vi "Host Main.vi"() -> ()   [LabVIEW 2021]
doc: "This application launches and executes the Tag Bus Data framework configuration for the specified target alias. This is a simple example of the framework API functions, but may also be a suitable starting point for a Host UI or Thick Client that is running a local version of the framework."
uses:
  <vilib>/NI/Module Execution Interface/Engine Runtime/Execution States.ctl
  <vilib>/NI/Module Execution Interface/Engine Runtime/Fault.ctl
  <vilib>/NI/Tag Bus Module Framework/runtime/error classification.ctl
  <vilib>/userdefined/High Color/nirio_resource_hc.ctl
  <vilib>/NI/Module Execution Interface/Engine Runtime/Engine Runtime Interface.lvclass
  <vilib>/NI/DCAF/Tag Editor Core/Framework Configuration Classes/target runtime/PL_Target Runtime.lvclass
  <vilib>/NI/Tag Bus Module Framework/FPGA manager/FPGA manager.lvlib
  <vilib>/rvi/interface/nirviOpenFPGA/nirviOpenFPGA.xnode
  <vilib>/NI/Tag Bus Module Framework/FPGA manager/methods.ctl
  <vilib>/NI/Tag Bus Module Framework/runtime/TBM module execution interface.lvclass
panel:
  in  "configuration file path":path=path "C:/Documentation/Trunk/Getting Started Material/Hands On/Hands-On_3/Excercises/Multiplexer/Multiplexer.pcfg"
  in  "target alias":string="PC"
  out "engine status":T4(array[cluster])
  in  "stop":bool
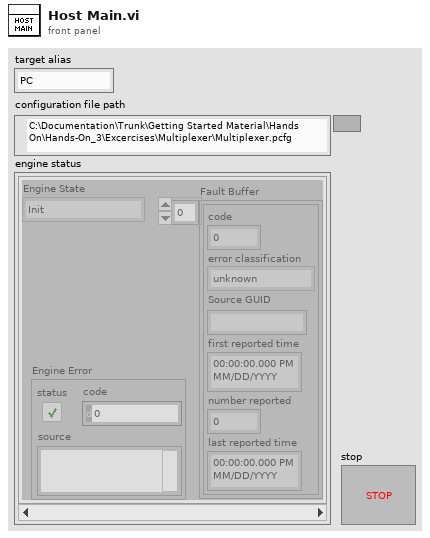
[diagram p1: front panel]
types:
  T1 = typedef "Engine Runtime Interface.lvclass/Execution States.ctl" = enum16{"Init", "Pre-Operational", "Safe-Operational", "Operational", "Stopped"}
  T2 = typedef "Engine Runtime Interface.lvclass/Fault.ctl" = cluster{"code":i32, "error classification":T3, "Source GUID":string, "first reported time":timestamp, "number reported":u32, "last reported time":timestamp}
  T3 = typedef "TBM module execution interface.lvclass/error classification.ctl" = enum16{"unknown", "none", "trivial", "recoverable", "critical"}
  T4 = cluster{"Engine State":T1, "Fault Buffer":T2[], "Engine Error":errorcluster}[]
  T5 = typedef "FPGA manager.lvlib/methods.ctl" = enum16{"initialize bitfile", "cache bitfile", "locate bitfile", "close bitfile", "clear manager"}
  T6 = typedef "nirio_resource_hc.ctl" = tag
  T7 = cluster{"Engine State":T1, "Fault Buffer":T2[], "Engine Error":errorcluster}
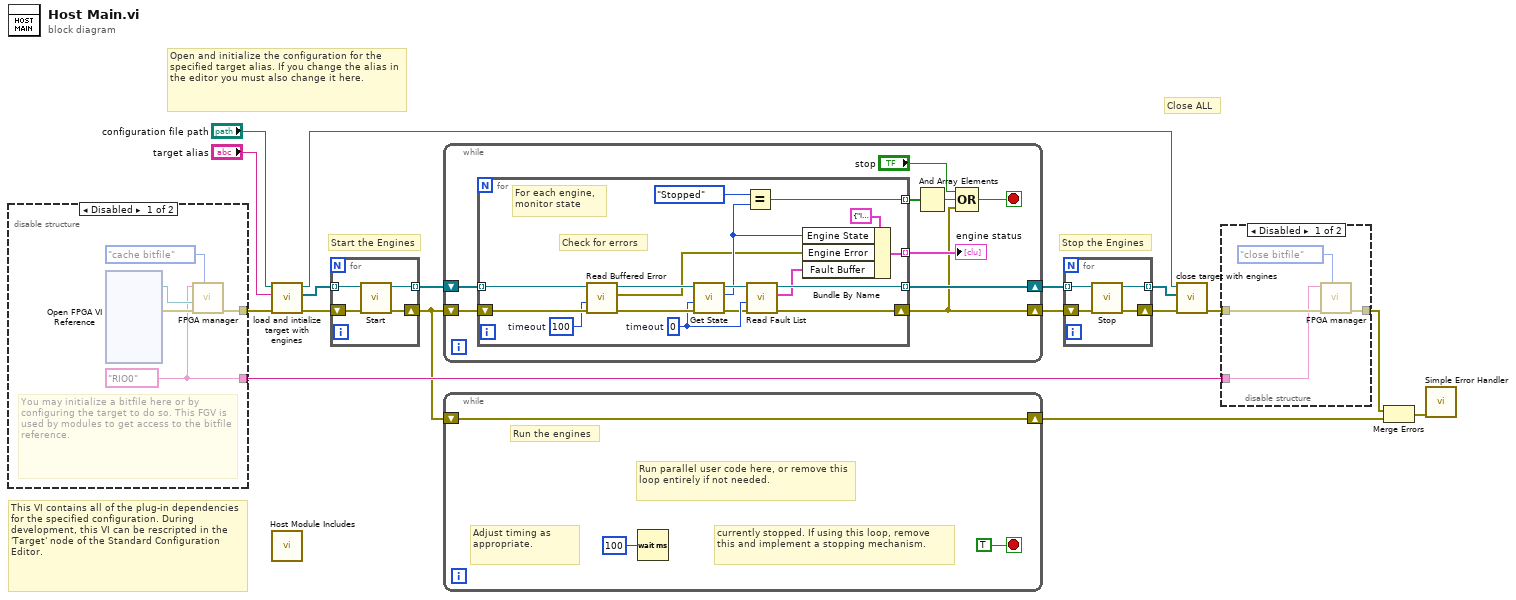
[diagram p0: block diagram]
diagram:
  # "Start the Engines"
  # "Open and initialize the configuration for the specified target alias. If you change the alias in the editor you must also change it here."
  # "Close ALL"
  # "Stop the Engines"
  # "This VI contains all of the plug-in dependencies for the specified configuration. During development, this VI can be rescripted in the 'Target' node of the Standard Configuration Editor."
  # "Run the engines"
  n1 = disable-structure shown="Disabled" {
    disable-tunnel: [w22 _] -> w7
    disable-tunnel: [w18 _] -> w6
    frame Disabled {
      w18 = T6 "RIO0" ("RIO resource")
      # "You may initialize a bitfile here or by configuring the target to do so. This FGV is used by modules to get access to the bitfile reference."
      n2 = xnode "Open FPGA VI Reference"() -> ("FPGA VI Reference Out"=w20:refnum<k20>, "error out"=w21:errorcluster)  [unwired: 2 in]
      n3 = call <vilib>:"FPGA manager.vi"("action"=methods."cache bitfile", "error in"=w21, "bitfile to cache"=w20, "RIO resource"=w18) -> ("error out"=w22:errorcluster)  [unwired: 5 in, 2 out]
    }
    frame Enabled {
    }
  }
  n4 = call <vilib>:"load and intialize target with engines.vi"("error in"=w7, "target alias"="target alias", "file path"="configuration file path") -> ("error out"=w14:errorcluster, "engine runtime interfaces"=w13:refnum<class "Engine Runtime Interface.lvclass">[], "target runtime"=w10:refnum<class "PL_Target Runtime.lvclass">)  [unwired: 6 in]
  n5 = call "Host Module Includes.vi"() -> ()  [unwired: 12 in]
  n6 = for {
    tunnel: [w26] -> w17 mode=indexing
    tunnel: w13 -> [w23] mode=indexing
    shift-right: [w25] -> w5
    shift-left: w14 -> [w24]
    n7 = call-dynamic "Start.vi"("error in"=w24, "Engine Runtime Interface in"=w23) -> ("error out"=w25:errorcluster, "Engine Runtime Interface out"=w26:refnum<class "Engine Runtime Interface.lvclass">)  [unwired: 8 in]
  }
  n8 = while {
    shift-right: [w33] -> w16
    shift-left: w17 -> [w35]
    shift-right: [w27] -> w15
    shift-left: w5 -> [w34]
    stop <- w31 stop-if-true
    n9 = for {
      tunnel: w35 -> [w52] mode=indexing
      tunnel: [w44] -> w33 mode=indexing
      tunnel: [w47] -> w29 mode=indexing
      shift-right: [w43] -> w27
      shift-left: w34 -> [w51]
      tunnel: [w39] -> w30 mode=indexing
      w42 = 0  # timeout
      w46 = 100  # timeout
      # "For each engine, \nmonitor state"
      # "Check for errors"
      n10 = call-dynamic "Read Buffered Error.vi"("error in"=w51, "timeout in ms (0)"=w46, "Engine Runtime Interface in"=w52) -> ("error out"=w49:errorcluster, "Engine Error"=w37:errorcluster, "Engine Runtime Interface out"=w50:refnum<class "Engine Runtime Interface.lvclass">)  [unwired: 6 in]
      n11 = call-dynamic "Get State.vi"("error in"=w49, "timeout (-1)"=w42, "Engine Runtime Interface in"=w50) -> ("error out"=w36:errorcluster, "Engine State"=w41:T1, "Engine Runtime Interface out"=w45:refnum<class "Engine Runtime Interface.lvclass">)  [unwired: 6 in]
      n12 = Equal?(x=Execution_States."Stopped" ("Engine State"), y=w41) -> (x = y?=w47:bool)
      n13 = call-dynamic "Read Fault List.vi"("error in"=w36, "timeout (-1)"=w42, "Engine Runtime Interface in"=w45) -> ("error out"=w43:errorcluster, "faults"=w40:T2[], "Engine Runtime Interface out"=w44:refnum<class "Engine Runtime Interface.lvclass">)  [unwired: 6 in]
      n14 = Bundle By Name(cluster=T7 {"Engine State"=enum."Init", "Fault Buffer"=[], "Engine Error"={"status"=FALSE, "code"=0, "source"=""}}, "Engine State"=w41, "Engine Error"=w37, "Fault Buffer"=w40) -> (w39:T7)
    }
    "engine status" <- w30
    n15 = And Array Elements(Boolean array=w29) -> (logical AND=w28:bool)
    n16 = Compound Arithmetic op=OR("stop", w28, w27) -> (w31:bool)
  }
  n17 = while {
    shift-right: [w53] -> w4
    shift-left: w5 -> [w53]
    stop <- TRUE stop-if-true
    # "currently stopped. If using this loop, remove \nthis and implement a stopping mechanism."
    # "Adjust timing as appropriate."
    # "Run parallel user code here, or remove this loop entirely if not needed."
    n18 = Wait (ms)(milliseconds to wait=u32 100) -> ()  [unwired: 1 out]
  }
  n19 = for {
    tunnel: w16 -> [w59] mode=indexing
    shift-right: [w56] -> w9
    shift-left: w15 -> [w58]
    tunnel: [w57] -> w11 mode=indexing
    n20 = call-dynamic "Stop.vi"("error in"=w58, "Engine Runtime Interface in"=w59) -> ("error out"=w56:errorcluster, "Engine Runtime Interface out"=w57:refnum<class "Engine Runtime Interface.lvclass">)  [unwired: 8 in]
  }
  n21 = call <vilib>:"close target with engines.vi"("error in"=w9, "Engine Runtime Interfaces"=w11, "Target Runtime"=w10) -> ("error out"=w3:errorcluster)  [unwired: 8 in]
  n22 = disable-structure shown="Disabled" {
    disable-tunnel: [w62 w64] -> w2
    disable-tunnel: w3 -> [w63 w64]
    disable-tunnel: w6 -> [w60 _]
    frame Disabled {
      n23 = call <vilib>:"FPGA manager.vi"("action"=methods."close bitfile", "error in"=w63, "RIO resource"=w60) -> ("error out"=w62:errorcluster)  [unwired: 6 in, 2 out]
    }
    frame Enabled {
    }
  }
  n24 = Merge Errors(w2, w4) -> (w1:errorcluster)
  n25 = call <vilib>:"Simple Error Handler.vi"("error in (no error)"=w1) -> ()  [unwired: 4 in, 5 out]
